vi "FTDI SPI GPIO Set.vi"(4 "nCS":u8 max=4 step=1, 5 "ClockRate":u32=50000, 6 "Relays (1-10)":bool[](array[boolean])=[FALSE, FALSE, FALSE, FALSE, FALSE, FALSE, FALSE, FALSE, FALSE, FALSE], 7 "Mode":T1(ring), 8 "Use Extra":bool, 9 "Channel Decimal":u16 max=10, 10 "Addr":T2 items=["Addr-0", "Addr-1", "Addr-2", "Addr-3", "Addr-4", "Addr-5", "Addr-6", "Addr-7"], 11 "Handler In":u32) -> (0 "error out":errorcluster, 1 "LATCH Reg":u16, 2 "OK":bool, 3 "Handler Out":u32)   [LabVIEW 2018]
uses:
  PROJEKT/NIKO/Labview/Niko V4/FTDI SPI/Ctl/Sub Addr.ctl
panel:
  out "Latch 0":u16
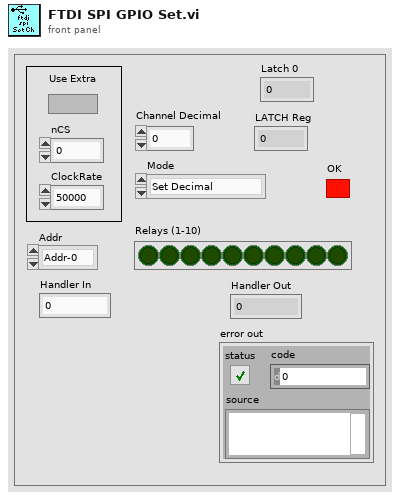
[diagram p1: front panel]
types:
  T1 = enum16{"Set Decimal", "Set Binary", "Set Channels", "Reset Channels", "Togle Channel"}
  T2 = typedef "Sub Addr.ctl" = u16
  T3 = cluster{"ClockRate":u32, "LatencyTimer":u8, "configOptions 24-31":i8, "configOptions 16-23":i8, "configOptions 8-15":i8, "configOptions 0-7":u32, "Pin":u32, "reserved":u16}
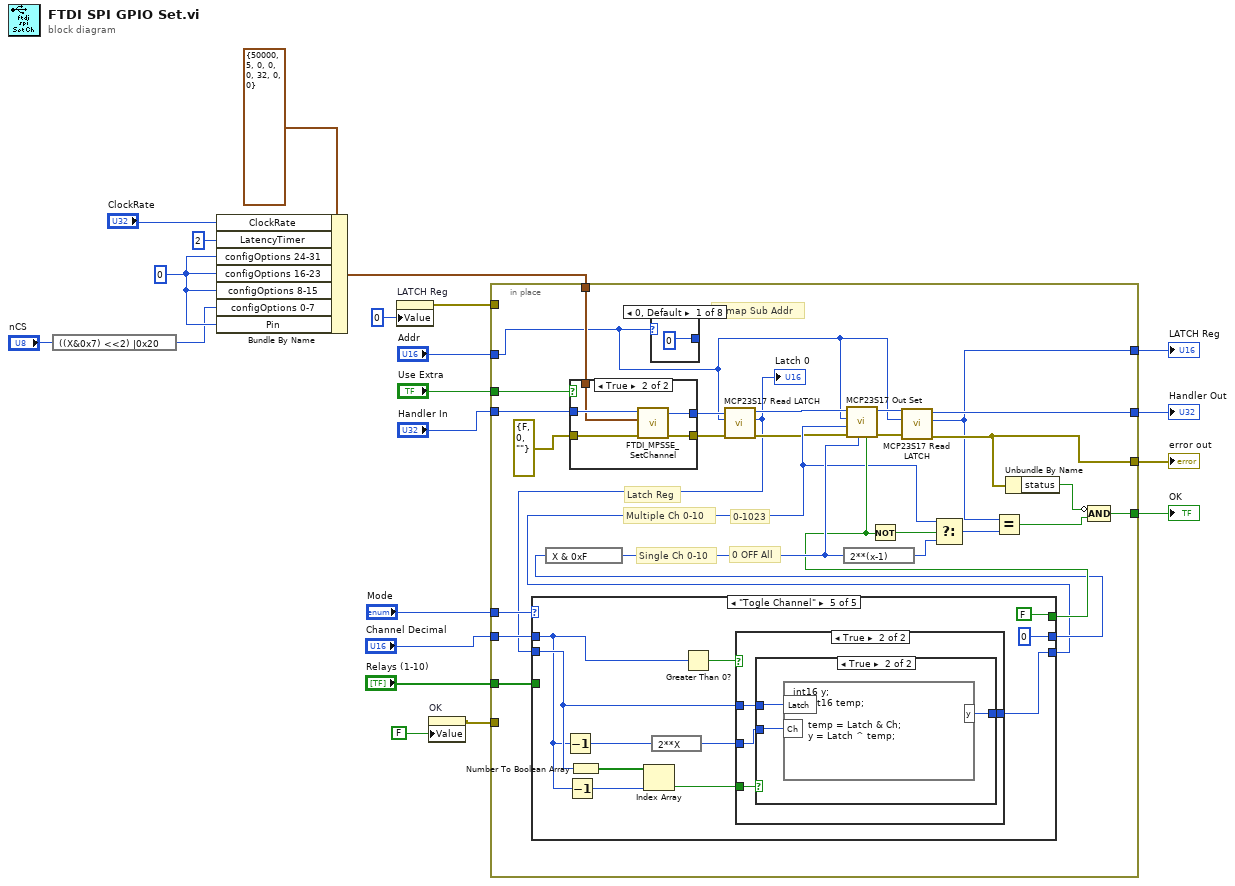
[diagram p0: block diagram]
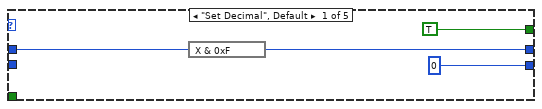
[diagram p2: hidden frame]
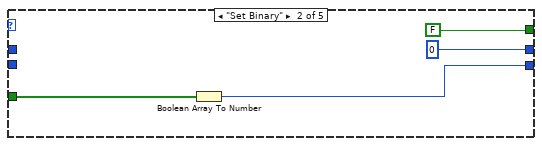
[diagram p3: hidden frame]
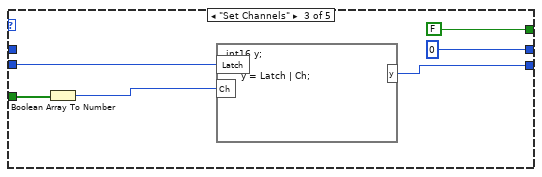
[diagram p4: hidden frame]
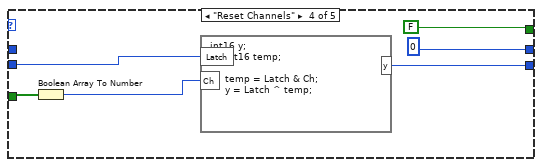
[diagram p5: hidden frame]
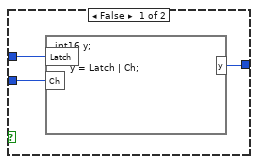
[diagram p7: hidden frame]
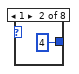
[diagram p8: hidden frame]
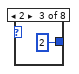
[diagram p9: hidden frame]
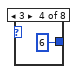
[diagram p10: hidden frame]
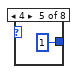
[diagram p11: hidden frame]
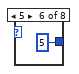
[diagram p12: hidden frame]
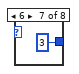
[diagram p13: hidden frame]
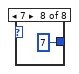
[diagram p14: hidden frame]
diagram:
  w9 = i8 0 ("configOptions 16-23")
  n1 = expression code="((X&0x7) <<2) |0x20"("nCS") -> (w6:u8)
  n2 = Bundle By Name(cluster=T3 {"ClockRate"=50000, "LatencyTimer"=5, "configOptions 24-31"=0, "configOptions 16-23"=0, "configOptions 8-15"=0, "configOptions 0-7"=32, "Pin"=0, "reserved"=0} ("config"), "ClockRate"="ClockRate", "LatencyTimer"=u8 2, "configOptions 24-31"=w9, "configOptions 16-23"=w9, "configOptions 8-15"=w9, "configOptions 0-7"=w6, "Pin"=w9) -> (w12:T3)
  n3 = property on="LATCH Reg" class="DigNum (strict)"("Value"=u16 0 ("LATCH Reg")) -> (error out=w15:errorcluster)  [unwired: 2 in, 1 out]
  n4 = property on="OK" class="Bool (strict)"("Value"=FALSE ("OK")) -> (error out=w5:errorcluster)  [unwired: 2 in, 1 out]
  n5 = in-place {
    in-place-border: [w49] -> w21
    in-place-border: [w48] -> w20
    in-place-border: "Handler In" -> [w41]
    in-place-border: [w46] -> w18
    in-place-border: [w47] -> w17
    in-place-border: "Addr" -> [w22]
    in-place-border: w15 -> [_]
    in-place-border: w12 -> [w40]
    in-place-border: w5 -> [_]
    in-place-border: "Mode" -> [w34]
    in-place-border: "Channel Decimal" -> [w33]
    in-place-border: "Relays (1-10)" -> [w32]
    in-place-border: "Use Extra" -> [w24]
    # "Latch Reg"
    # "Multiple Ch 0-10"
    # "Remap Sub Addr"
    # "0 OFF All"
    # "Single Ch 0-10"
    # "0-1023"
    n6 = case shown="True" w24 {
      tunnel: w41 -> [w101 w104]
      tunnel: [w101 w105] -> w27
      tunnel: [w100 w106] -> w28
      tunnel: errorcluster {"status"=FALSE, "code"=0, "source"=""} ("error constant") -> [w100 w102]
      tunnel: w40 -> [_ w103]
      frame False {
      }
      frame True {
        n7 = call "FTDI_MPSSE_SetChannel.vi"("error in (no error)"=w102, "config"=w103, "handle"=w104) -> ("error out"=w106:errorcluster, "handle out"=w105:u32)  [unwired: 7 in]
      }
    }
    n8 = case shown="0, Default" w22 {
      tunnel: [0 4 2 6 1 5 3 7] -> _
      frame 0, Default {
      }
      frame 1 {
      }
      frame 2 {
      }
      frame 3 {
      }
      frame 4 {
      }
      frame 5 {
      }
      frame 6 {
      }
      frame 7 {
      }
    }
    n9 = call "MCP23S17 Read LATCH.vi"("error in (no error)"=w28, "Addr"=w22, "handle"=w27) -> ("error out"=w25:errorcluster, "LATCH"=w23:u16, "handle out"=w26:u32)  [unwired: 4 in, 2 out]
    "Latch 0" <- w23
    n10 = case shown="\"Togle Channel\"" w34 {
      tunnel: [TRUE FALSE FALSE FALSE FALSE] -> w31
      tunnel: w33 -> [w52 _ _ _ w71]
      tunnel: [w51 u16 0 ("Channel Decimal") u16 0 ("Channel Decimal") u16 0 ("Channel Decimal") u16 0 ("Channel Decimal")] -> w30
      tunnel: [u32 0 w55 w60 w66 w75] -> w29
      tunnel: w32 -> [_ w54 w61 w64 _]
      tunnel: w23 -> [_ _ w59 w67 w78]
      frame "Set Decimal", Default {
        n11 = expression code="X & 0xF"(w52) -> (w51:u16)
      }
      frame "Set Binary" {
        n12 = Boolean Array To Number(Boolean array=w54) -> (number=w55:u32)
      }
      frame "Set Channels" {
        n13 = Boolean Array To Number(Boolean array=w61) -> (number=w58:u32)
        n14 = formula code="int16 y;\n\n     y = Latch | Ch;"("Latch"=w59, "Ch"=w58) -> ("y"=w60:i16)
      }
      frame "Reset Channels" {
        n15 = Boolean Array To Number(Boolean array=w64) -> (number=w65:u32)
        n16 = formula code="int16 y;\n     int16 temp;\n\n     temp = Latch & Ch;\n     y = Latch ^ temp;"("Latch"=w67, "Ch"=w65) -> ("y"=w66:i16)
      }
      frame "Togle Channel" {
        n17 = Decrement(x=w71) -> (x-1=w73:u16)
        n18 = Decrement(x=w71) -> (x-1=w76:u16)
        n19 = Number To Boolean Array(number=w78) -> (Boolean array=w77:bool[])
        n20 = Index Array(array=w77, index=w76) -> (element=w79:bool)
        n21 = expression code="2**X"(w73) -> (w72:u16)
        n22 = Greater Than 0?(x=w71) -> (x > 0?=w70:bool)
        n23 = case shown="True" w70 {
          tunnel: w79 -> [_ w85]
          tunnel: w78 -> [w81 w84]
          tunnel: [w81 w83] -> w75
          tunnel: w72 -> [_ w82]
          frame False {
          }
          frame True {
            n24 = case shown="True" w85 {
              tunnel: [w88 w91] -> w83
              tunnel: w84 -> [w87 w90]
              tunnel: w82 -> [w86 w89]
              frame False {
                n25 = formula code="int16 y;\n\n     y = Latch | Ch;"("Latch"=w87, "Ch"=w86) -> ("y"=w88:i16)
              }
              frame True {
                n26 = formula code="int16 y;\n     int16 temp;\n\n     temp = Latch & Ch;\n     y = Latch ^ temp;"("Latch"=w90, "Ch"=w89) -> ("y"=w91:i16)
              }
            }
          }
        }
      }
    }
    n27 = expression code="X & 0xF"(w30) -> (w35:u16)
    n28 = expression code="2**(x-1)"(w35) -> (w43:u16)
    n29 = call "MCP23S17 Out Set.vi"("SW Mode"=w31, "Set Single Ch"=w35, "error in (no error)"=w25, "Channels"=w29, "Addr"=w22, "handle"=w26) -> ("error out"=w38:errorcluster, "handle out"=w37:u32)  [unwired: 4 in]
    n30 = Not(x=w31) -> (.not. x?=w42:bool)
    n31 = call "MCP23S17 Read LATCH.vi"("error in (no error)"=w38, "Addr"=w22, "handle"=w37) -> ("error out"=w48:errorcluster, "LATCH"=w47:u16, "handle out"=w49:u32)  [unwired: 4 in, 2 out]
    n32 = Select(t=w29, s=w42, f=w43) -> (s? t:f=w44:u32)
    n33 = Equal?(x=w47, y=w44) -> (x = y?=w36:bool)
    n34 = Unbundle By Name(w48) -> ("status"=w45:bool)
    n35 = Compound Arithmetic op=AND(invert w45, w36) -> (w46:bool)
  }
  "Handler Out" <- w21
  "error out" <- w20
  "OK" <- w18
  "LATCH Reg" <- w17
